vi "cw_1_5.vi"() -> ()   [LabVIEW 2022 SP3]
panel:
  out "U32":u32
  out "U8":u8
  out "U8":u8
  in  "I8":i8
  in  "U32":u32
  in  "I32":i32
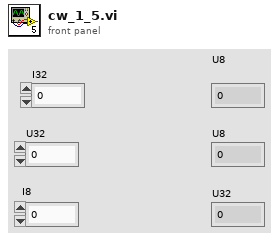
[diagram p1: front panel]
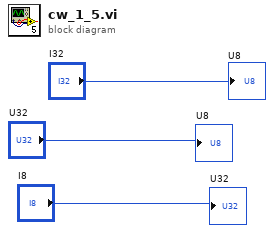
[diagram p0: block diagram]
diagram:
  "U8" <- "I32"
  "U8" <- "U32"
  "U32" <- "I8"
